vi "MainForKeithley.vi"() -> ()   [LabVIEW 2018]
uses:
  classes/Tushars Events Toolkit/Software/Modules/EventClient_ObjectReference.ctl
  classes/Variable Manager/VariableManager_Bool.vi
  classes/Variable Manager/VariableManager_Double.vi
  <vilib>/Utility/file.llb/Write To Spreadsheet File (string).vi
  classes/Variable Manager/VariableManager_String.vi
  Strict Type Controls/Command.ctl
panel:
  out "filterSetup?":bool
  out "Quit":bool
  out "error out":errorcluster
  in  "error in (no error)":errorcluster
  in  "abort":bool
  in  "start":bool
  out "gratSetup?":bool
  out "statusFilter":bool
  in  "Start Filter":bool
  out "Agilent Current":dbl format="%#.4f A"
  out "Agilent Voltage":dbl format="%#.4f V"
  out "Test Status":bool
  out "statusMerlin":bool
  out "statusMC":bool
  out "statusPS":bool
  out "statusSM":bool
  in  "Start Merlin":bool
  in  "Start Monochromator":bool
  in  "Start Power Supply":bool
  in  "Start Source Meter":bool
  out "Merlin Voltage":dbl format="%#.7f mV"
  out "Measuring Wavelength":dbl format="%#.7f nm"
  out "Source Meter Voltage":dbl format="%#.7f mV"
  in  "tab":T1(tab)=enum."Script"
  in  "exportVT":bool
  out "VTGraph":cluster{dbl[], dbl[]}(graph)
  in  "Test Mode":enum16{"Time Mode", "dV/dt Mode"}(ring)
  in  "Log Interval":u32=50 min=100 step=1 format="%.0f mSec"
  in  "Test Time":dbl step=1.0 format="%<%H:%M:%S>t"
  out "Time Remaining":dbl format="%<%H:%M:%S>t"
  in  "Target dV/dt":dbl format="%#.9f mV"
  in  "Lock In time":dbl step=1.0 format="%<%H:%M:%S>t"
  out "dV/dt":dbl format="%#.11f mV"
  out "Locked Time":dbl step=1.0 format="%<%H:%M:%S>t"
  in  "Perform Test After":T1(ring)=enum."Voltage Vs Wavelength"
  in  "Frequency":u32=8 min=8 max=1100 step=1
  in  "setOffsets":bool
  in  "portD":bool
  in  "portA":bool
  in  "Settling Time (ms)":dbl=5000.0
  in  "To":dbl=1000.0
  in  "Step":dbl=100.0
  in  "From":dbl=100.0
  in  "exportSweep":bool
  out "sweep":cluster{dbl[], dbl[]}[](graph)
  in  "SetSlit":bool
  in  "SetGrating":bool
  in  "setWavelength":bool
  in  "Wavelength":dbl
  in  "Slit":string(combo)
  in  "GratingNo":u8=1 min=1 max=3 step=1
  in  "setMerlin":bool
  in  "#Filter Stages":enum16{"None", "1 Pole", "2 Pole"}(ring)
  in  "Phase":enum16{"1 Phase", "2 Phase"}(ring)
  in  "SyncMode":T2(ring)
  in  "Time Const":T3(ring)
  in  "Sweep Results":i32(listbox)
  in  "tabOnScript":enum32{"V Vs Time", "V Vs Wavelength"}(tab)
  out "scriptGraph":cluster{dbl[], dbl[]}(graph)
  in  "exportScriptResults":bool
  out "scriptSweep":cluster{dbl[], dbl[]}[](graph)
  in  "exportScriptWave":bool
  in  "Command":T4
  in  "Parm 4":dbl format="%#.6f"
  in  "Parm 3":dbl format="%#.6f"
  in  "openScript":bool
  in  "exportScript":bool
  in  "update":bool
  in  "Parm 2":dbl format="%#.6f"
  in  "Parm 1":dbl format="%#.6f"
  in  "script":i32(listbox)
  in  "add":bool
  in  "remove":bool
  in  "Script Avg Interval":u32=200 min=100 step=1 format="%.0f mSec"
  # "Status"
  # "Test Type"
  # "Test Time"
  # "Voltage Results"
  # "Monochromator"
  # "Sweep"
  # "NOTE:\n1. if this LED is OFF then GPIB is not connected...\n2. Close program before power off Instruments..."
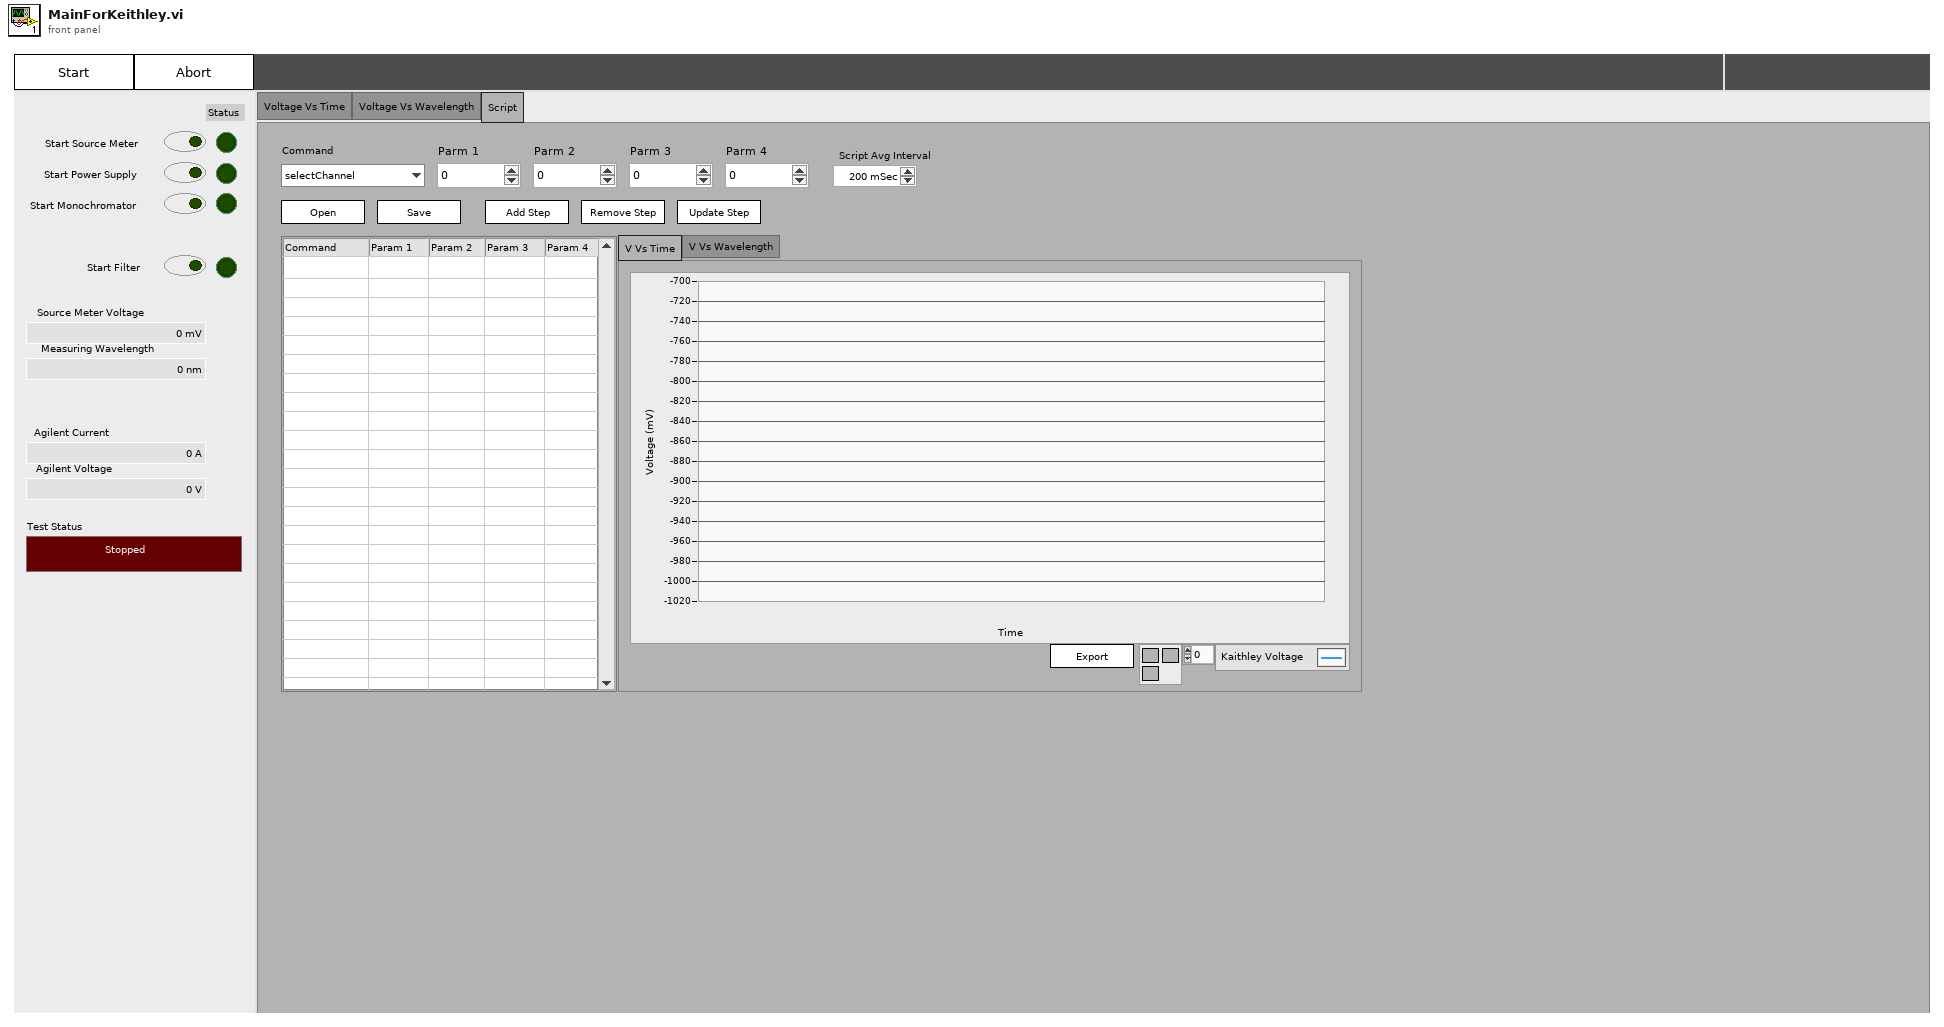
[diagram p1: front panel]
types:
  T1 = enum32{"Voltage Vs Time", "Voltage Vs Wavelength", "Script"}
  T2 = enum16{"Int Chop Off", "Int Chop On", "Ext Chop Off", "Ext Chop On"}
  T3 = enum16{".003s", ".010s", ".030s", ".100s", ".300s", "1.00s", "3.00s", "10.0s", "30.0s", "100s"}
  T4 = typedef "Command.ctl" = enum16{"selectChannel", "setDCVoltage", "setDCCurrent", "setVoltageSteps", "wait", "setWavelength", "setWavelengthSteps"}
  T5 = enum32{"invalid app kind", "Development System", "Run Time System", "Student Edition", "Embedded LabVIEW", "Evaluation", "Custom"}
  T6 = cluster{"startTime":u32, "lastUpdate":u32, "lastVoltage":dbl, "run?":bool, "From":dbl, "time":dbl[], "MerlinVal":dbl[], "SMVolt":dbl[], "sweepType":enum16{"ASC", "DESC"}, "Wavlnth":dbl[], "Test Mode":enum16{"Time Mode", "dV/dt Mode"}, "tab":enum32{"Voltage Vs Time", "Voltage Vs Wavelength", "Script"}, "script":string[][], "dV/dt":dbl[], "graphUpdate":u32}
  T7 = typedef "EventClient_ObjectReference.ctl" = refnum<k1>
  T8 = cluster{"#Stages":enum16{"None", "1 Pole", "2 Pole"}, "Phase":enum16{"1 Phase", "2 Phase"}, "SyncMode":enum16{"Int Chop Off", "Int Chop On", "Ext Chop Off", "Ext Chop On"}, "Time Const":enum16{".003s", ".010s", ".030s", ".100s", ".300s", "1.00s", "3.00s", "10.0s", "30.0s", "100s"}, "Frequency":u32}
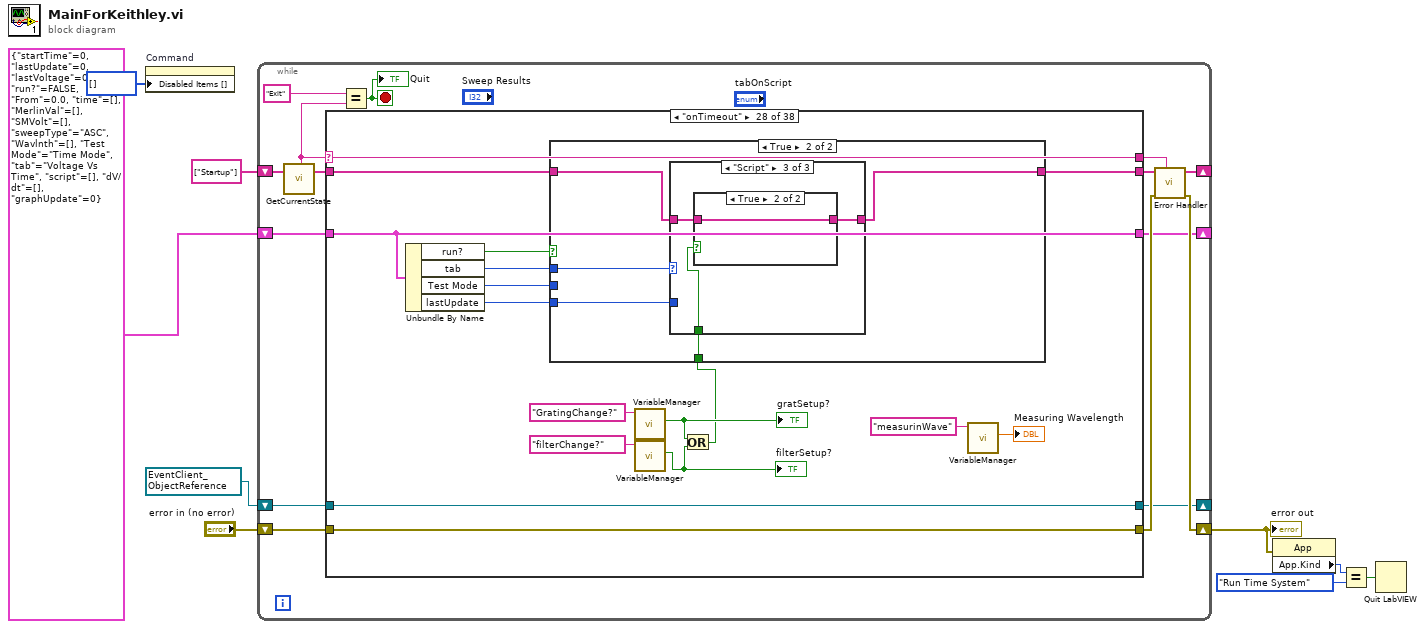
[diagram p0: block diagram]
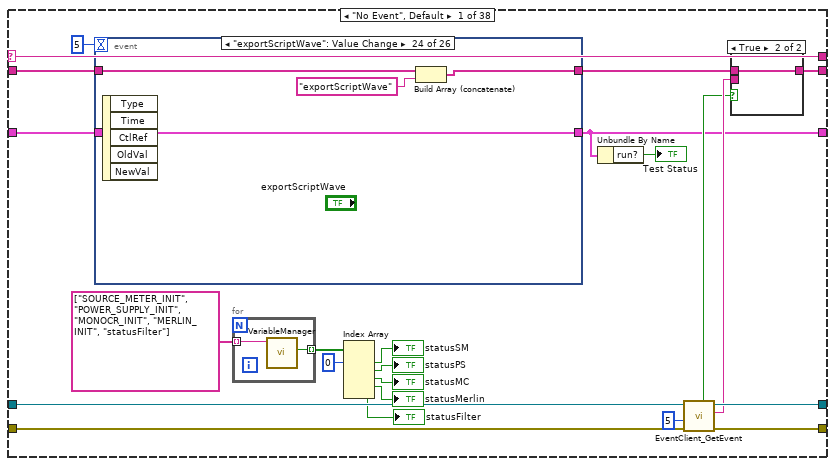
[diagram p2: hidden frame]
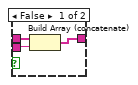
[diagram p3: hidden frame]
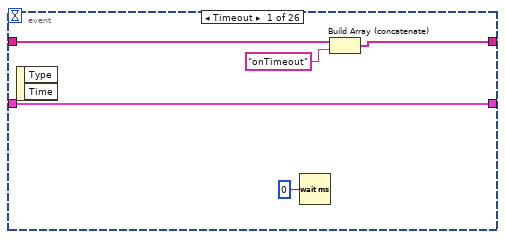
[diagram p4: hidden frame]
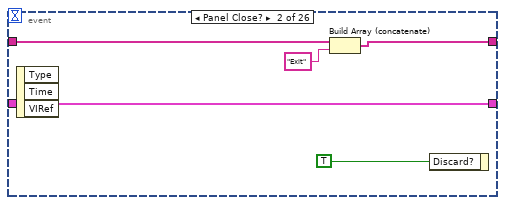
[diagram p5: hidden frame]
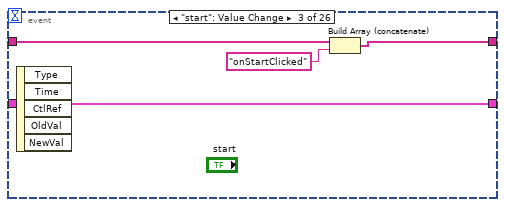
[diagram p6: hidden frame]
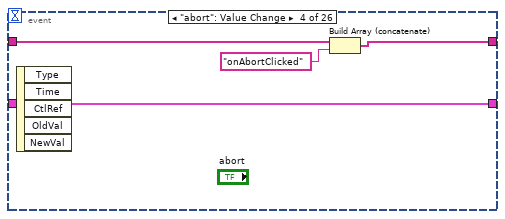
[diagram p7: hidden frame]
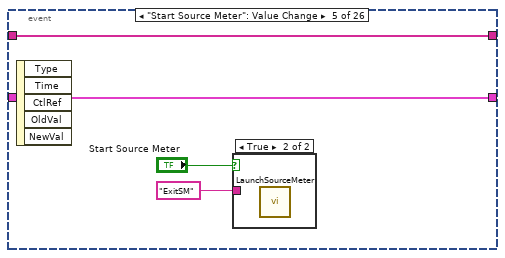
[diagram p8: hidden frame]
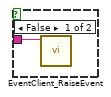
[diagram p9: hidden frame]
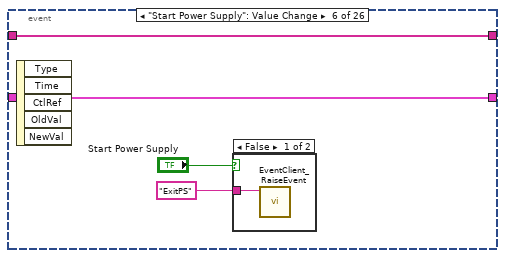
[diagram p10: hidden frame]
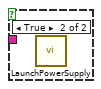
[diagram p11: hidden frame]
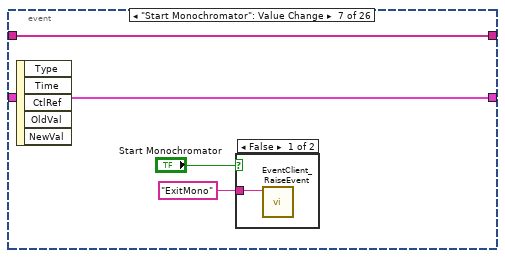
[diagram p12: hidden frame]
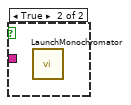
[diagram p13: hidden frame]
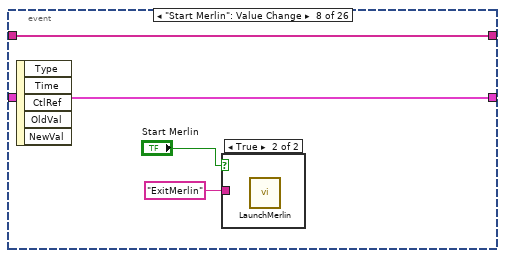
[diagram p14: hidden frame]
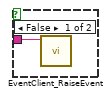
[diagram p15: hidden frame]
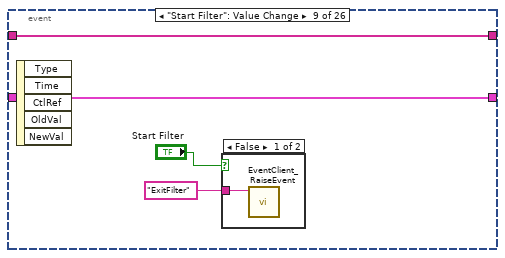
[diagram p16: hidden frame]
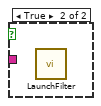
[diagram p17: hidden frame]
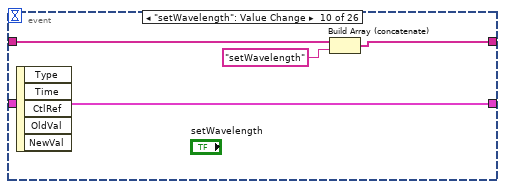
[diagram p18: hidden frame]
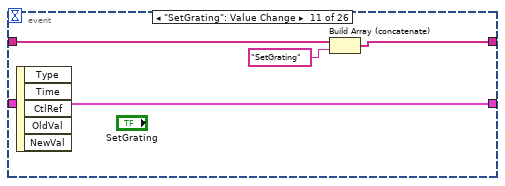
[diagram p19: hidden frame]
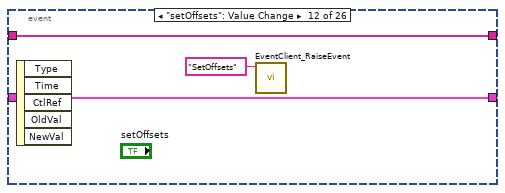
[diagram p20: hidden frame]
diagram:
  w8 = T7 refnum items=["EventClient"] ("reference")
  n1 = property on="Command" class="Enum (strict)"("Disabled Items []"=i32[] []) -> ()  [unwired: 2 in, 2 out]
  n2 = while {
    shift-right: [w20] -> _
    shift-left: string[] ["Startup"] ("State Array Out") -> [w24]
    shift-right: [w16] -> w5
    shift-left: "error in (no error)" -> [w17]
    shift-right: [w13] -> _
    shift-left: w8 -> [w12]
    shift-right: [w10] -> _
    shift-left: T6 {"startTime"=0, "lastUpdate"=0, "lastVoltage"=0.0, "run?"=FALSE, "From"=0.0, "time"=[], "MerlinVal"=[], "SMVolt"=[], "sweepType"=enum."ASC", "Wavlnth"=[], "Test Mode"=enum."Time Mode", "tab"=enum."Voltage Vs Time", "script"=[], "dV/dt"=[], "graphUpdate"=0} -> [w11]
    stop <- w21 stop-if-true
    n3 = call "GetCurrentState.vi"("State Array In"=w24) -> ("Current State"=w14:string, "State Array Out"=w23:string[])  [unwired: 17 in]
    n4 = case shown="\"onTimeout\"" w14 {
      selector: w14 -> [w47 w189 w198 w208 w226 w242 w265 w292 w310 w321 w342 w359 w367 w394 w410 w421 w433 w441 w445 w454 w463 w475 w483 w493 w522 w533 w538 w556 w608 w628 w658 w690 w715 w779 w834 w869 w898 w914]
      tunnel: w23 -> [w46 w188 w204 w209 w227 w243 w266 w293 w311 w322 w343 w360 w368 w395 w411 w422 w434 w442 w449 w458 w465 w479 w484 w494 w523 w534 w539 w547 w591 w612 w650 w682 w706 w780 w835 w870 w897 w901]
      tunnel: [w37 w187 w204 w209 w227 w243 w266 w293 w311 w322 w343 w360 w368 w395 w411 w422 w434 w442 w449 w458 w465 w479 w484 w494 w523 w534 w539 w548 w590 w611 w649 w684 w705 w780 w823 w870 w897 w901] -> w19
      tunnel: [w42 w181 w199 w207 w225 w241 w264 w291 w309 w320 w341 w358 w366 w393 w409 w420 w427 w435 w446 w455 w461 w476 w482 w489 w518 w529 w537 w555 w607 w627 w657 w689 w713 w761 w830 w868 w896 errorcluster {"status"=FALSE, "code"=0, "source"=""} ("error in (no error)")] -> w15
      tunnel: [w47 w189 w198 w208 w226 w242 w265 w292 w310 w321 w342 w359 w367 w394 w410 w421 w433 w441 w445 w454 w463 w475 w483 w493 w522 w533 w538 w556 w608 w628 w658 w690 w715 w779 w834 w869 w898 w914] -> w18
      tunnel: w17 -> [w43 w168 w202 w207 w225 w241 w264 w291 w309 w320 w341 w358 w366 w393 w409 w420 w428 w436 w447 w456 w460 w477 w482 w491 w520 w531 w537 w555 w607 w627 w657 w689 w713 w760 w831 w868 w896 w902]
      tunnel: [w41 w179 w201 w206 w224 w240 w263 w290 w308 w319 w340 w357 w365 w392 w408 w419 w432 w440 w448 w457 w464 w478 w481 w487 w516 w527 w536 w554 w606 w626 w656 w688 w714 w778 w833 w867 w895 w900] -> w13
      tunnel: w12 -> [w44 _ w203 w206 w224 w240 w263 w290 w308 w319 w340 w357 w365 w392 w408 w419 w432 w440 w448 w457 w464 w478 w481 w492 w521 w532 w536 w554 w606 w626 w656 w688 w714 w778 w833 w867 w895 w900]
      tunnel: w11 -> [w28 w177 w197 w205 w223 w239 w262 w289 w307 w318 w339 w356 w364 w391 w407 w418 w431 w439 w443 w453 w462 w468 w480 w485 w515 w526 w535 w553 w596 w625 w654 w687 w708 w777 w821 w860 w894 w899]
      tunnel: [w27 w177 w197 w205 w223 w239 w262 w289 w307 w318 w339 w356 w364 w390 w406 w418 w431 w439 w443 w453 w462 w468 w480 w485 w515 w526 w535 w553 w595 w622 w652 w687 w707 w776 w832 w859 w894 w899] -> w10
      frame "No Event", Default {
        n5 = event shown="[23] \"exportScriptWave\": Value Change" {
          selector: _ -> [_ _ _ _ _ _ _ _ _ _ _ _ _ _ _ _ _ _ _ _ _ _ _ _ _ _]
          dyn-events: _ -> [_ _ _ _ _ _ _ _ _ _ _ _ _ _ _ _ _ _ _ _ _ _ _ _ _ _]
          timeout: 5 -> [_ _ _ _ _ _ _ _ _ _ _ _ _ _ _ _ _ _ _ _ _ _ _ _ _ _]
          tunnel: [w56 w61 w66 w70 w75 w80 w85 w90 w95 w99 w103 w106 w110 w114 w118 w122 w126 w130 w134 w138 w142 w146 w150 w154 w158 w162] -> w38
          tunnel: w46 -> [w58 w63 w67 w71 w75 w80 w85 w90 w95 w100 w104 w106 w111 w115 w119 w123 w127 w131 w135 w139 w143 w147 w151 w155 w159 w163]
          tunnel: w28 -> [w57 w59 w64 w68 w74 w79 w84 w89 w94 w97 w101 w107 w108 w112 w116 w120 w124 w128 w132 w136 w140 w144 w148 w152 w156 w160]
          tunnel: [w57 w59 w64 w68 w74 w79 w84 w89 w94 w97 w101 w107 w108 w112 w116 w120 w124 w128 w132 w136 w140 w144 w148 w152 w156 w160] -> w27
          event Timeout {
            n6 = event-data() -> ()  [unwired: 1 in, 2 out]
            n7 = Wait (ms)(milliseconds to wait=u32 0) -> ()  [unwired: 1 out]
            n8 = Build Array (concatenate)(w58, "onTimeout" ("x")) -> (w56:string[])
          }
          event Panel Close? {
            n9 = event-data() -> ()  [unwired: 1 in, 3 out]
            n10 = Build Array (concatenate)(w63, "Exit" ("x")) -> (w61:string[])
            n11 = event-data("Discard?"=TRUE) -> ()  [unwired: 1 in, 1 out]
          }
          event "start": Value Change {
            n12 = event-data() -> ()  [unwired: 1 in, 5 out]
            n13 = Build Array (concatenate)(w67, "onStartClicked" ("x")) -> (w66:string[])
          }
          event "abort": Value Change {
            n14 = event-data() -> ()  [unwired: 1 in, 5 out]
            n15 = Build Array (concatenate)(w71, "onAbortClicked" ("x")) -> (w70:string[])
          }
          event "Start Source Meter": Value Change {
            n16 = event-data() -> ()  [unwired: 1 in, 5 out]
            n17 = case shown="True" "Start Source Meter" {
              tunnel: "ExitSM" -> [w76 _]
              frame False {
                n18 = call "EventClient_RaiseEvent.vi"("Event"=w76) -> ()  [unwired: 10 in, 1 out]
              }
              frame True {
                n19 = call "LaunchSourceMeter.vi"() -> ()  [unwired: 11 in, 1 out]
              }
            }
          }
          event "Start Power Supply": Value Change {
            n20 = event-data() -> ()  [unwired: 1 in, 5 out]
            n21 = case shown="False" "Start Power Supply" {
              tunnel: "ExitPS" -> [w81 _]
              frame False {
                n22 = call "EventClient_RaiseEvent.vi"("Event"=w81) -> ()  [unwired: 10 in, 1 out]
              }
              frame True {
                n23 = call "LaunchPowerSupply.vi"() -> ()  [unwired: 11 in, 1 out]
              }
            }
          }
          event "Start Monochromator": Value Change {
            n24 = event-data() -> ()  [unwired: 1 in, 5 out]
            n25 = case shown="False" "Start Monochromator" {
              tunnel: "ExitMono" -> [w86 _]
              frame False {
                n26 = call "EventClient_RaiseEvent.vi"("Event"=w86) -> ()  [unwired: 10 in, 1 out]
              }
              frame True {
                n27 = call "LaunchMonochromator.vi"() -> ()  [unwired: 11 in, 1 out]
              }
            }
          }
          event "Start Merlin": Value Change {
            n28 = event-data() -> ()  [unwired: 1 in, 5 out]
            n29 = case shown="True" "Start Merlin" {
              tunnel: "ExitMerlin" -> [w91 _]
              frame False {
                n30 = call "EventClient_RaiseEvent.vi"("Event"=w91) -> ()  [unwired: 10 in, 1 out]
              }
              frame True {
                n31 = call "LaunchMerlin.vi"() -> ()  [unwired: 11 in, 1 out]
              }
            }
          }
          event "Start Filter": Value Change {
            n32 = event-data() -> ()  [unwired: 1 in, 5 out]
            n33 = case shown="False" "Start Filter" {
              tunnel: "ExitFilter" -> [w96 _]
              frame False {
                n34 = call "EventClient_RaiseEvent.vi"("Event"=w96) -> ()  [unwired: 10 in, 1 out]
              }
              frame True {
                n35 = call "LaunchFilter.vi"() -> ()  [unwired: 11 in, 1 out]
              }
            }
          }
          event "setWavelength": Value Change {
            n36 = event-data() -> ()  [unwired: 1 in, 5 out]
            n37 = Build Array (concatenate)(w100, "setWavelength" ("x")) -> (w99:string[])
          }
          event "SetGrating": Value Change {
            n38 = event-data() -> ()  [unwired: 1 in, 5 out]
            n39 = Build Array (concatenate)(w104, "SetGrating" ("x")) -> (w103:string[])
          }
          event "setOffsets": Value Change {
            n40 = event-data() -> ()  [unwired: 1 in, 5 out]
            n41 = call "EventClient_RaiseEvent.vi"("Event"="SetOffsets") -> ()  [unwired: 10 in, 1 out]
          }
          event "SetSlit": Value Change {
            n42 = event-data() -> ()  [unwired: 1 in, 5 out]
            n43 = Build Array (concatenate)(w111, "SetSlit" ("x")) -> (w110:string[])
          }
          event "setMerlin": Value Change {
            n44 = event-data() -> ()  [unwired: 1 in, 5 out]
            n45 = Build Array (concatenate)(w115, "setMerlin" ("x")) -> (w114:string[])
          }
          event "exportSweep": Value Change {
            n46 = event-data() -> ()  [unwired: 1 in, 5 out]
            n47 = Build Array (concatenate)(w119, "exportSweep" ("x")) -> (w118:string[])
          }
          event "exportVT": Value Change {
            n48 = event-data() -> ()  [unwired: 1 in, 5 out]
            n49 = Build Array (concatenate)(w123, "exportVT" ("x")) -> (w122:string[])
          }
          event "portA": Value Change {
            n50 = event-data() -> ()  [unwired: 1 in, 5 out]
            n51 = Build Array (concatenate)(w127, "portA" ("x")) -> (w126:string[])
          }
          event "portD": Value Change {
            n52 = event-data() -> ()  [unwired: 1 in, 5 out]
            n53 = Build Array (concatenate)(w131, "portD" ("x")) -> (w130:string[])
          }
          event "add": Value Change {
            n54 = event-data() -> ()  [unwired: 1 in, 5 out]
            n55 = Build Array (concatenate)(w135, "addStep" ("x")) -> (w134:string[])
          }
          event "remove": Value Change {
            n56 = event-data() -> ()  [unwired: 1 in, 5 out]
            n57 = Build Array (concatenate)(w139, "removeStep" ("x")) -> (w138:string[])
          }
          event "update": Value Change {
            n58 = event-data() -> ()  [unwired: 1 in, 5 out]
            n59 = Build Array (concatenate)(w143, "updateStep" ("x")) -> (w142:string[])
          }
          event "exportScript": Value Change {
            n60 = event-data() -> ()  [unwired: 1 in, 5 out]
            n61 = Build Array (concatenate)(w147, "exportScript" ("x")) -> (w146:string[])
          }
          event "exportScriptResults": Value Change {
            n62 = event-data() -> ()  [unwired: 1 in, 5 out]
            n63 = Build Array (concatenate)(w151, "exportScriptResults" ("x")) -> (w150:string[])
          }
          event "exportScriptWave": Value Change {
            n64 = event-data() -> ()  [unwired: 1 in, 5 out]
            n65 = Build Array (concatenate)(w155, "exportScriptWave" ("x")) -> (w154:string[])
          }
          event "openScript": Value Change {
            n66 = event-data() -> ()  [unwired: 1 in, 5 out]
            n67 = Build Array (concatenate)(w159, "openScript" ("x")) -> (w158:string[])
          }
          event "script": Value Change {
            n68 = event-data() -> ()  [unwired: 1 in, 5 out]
            n69 = Build Array (concatenate)(w163, "onScriptRowSelected" ("x")) -> (w162:string[])
          }
        }
        n70 = for {
          tunnel: string[] ["SOURCE_METER_INIT", "POWER_SUPPLY_INIT", "MONOCR_INIT", "MERLIN_INIT", "statusFilter"] ("State Array Out") -> [w49] mode=indexing
          tunnel: [w48] -> w34 mode=indexing
          n71 = call-poly "VariableManager.vi"("Tag"=w49) -> ("Value out"=w48:bool)  [unwired: 7 in, 3 out]
        }
        n72 = Index Array(array=w34, index #1=0 ("index")) -> (element #1=→"statusSM":bool, element #2=→"statusPS":bool, element #3=→"statusMC":bool, element #4=→"statusMerlin":bool, element #5=→"statusFilter":bool)  [unwired: 4 in]
        n73 = Unbundle By Name(w27) -> ("run?"=→"Test Status":bool)
        n74 = call "EventClient_GetEvent.vi"("error in (no error)"=w43, "timeout in ms (-1)"=5, "reference"=w44) -> ("error out"=w42:errorcluster, "Name"=w40:string, "reference out"=w41:T7, "timed out?"=w39:bool)  [unwired: 4 in, 1 out]
        n75 = case shown="True" w39 {
          tunnel: w38 -> [w52 w53]
          tunnel: w40 -> [w51 _]
          tunnel: [w50 w53] -> w37
          frame False {
            n76 = Build Array (concatenate)(w52, w51) -> (w50:string[])
          }
          frame True {
          }
        }
      }
      frame "Startup" {
        w166 = cluster{dbl[], dbl[]}[] [] ("sweep")
        w167 = cluster{dbl[], dbl[]} {[], []} ("VTGraph")
        w171 = string[] ["Command", "Param 1", "Param 2", "Param 3", "Param 4"]  # script
        w172 = FALSE ("Start Source Meter")
        w165 = u32 200 ("Log Interval")
        # "If Multiple instnances of this VI are possible \nthen make sure that client created in each instance gets a different Name"
        n77 = local write "Log Interval"(w165) -> ()
        n78 = local write "Target dV/dt"(1.0 ("Target dV/dt")) -> ()
        n79 = local write "Lock In time"(30.0 ("Lock In time")) -> ()
        n80 = local write "sweep"(w166) -> ()
        n81 = local write "Test Time"(90.0 ("Locked Time")) -> ()
        n82 = local write "VTGraph"(w167) -> ()
        n83 = local write "scriptGraph"(w167) -> ()
        n84 = local write "Script Avg Interval"(w165) -> ()
        n85 = disable-structure shown="Disabled" {
          disable-tunnel: [w196 _] -> w173
          disable-tunnel: w168 -> [w195 _]
          frame Disabled {
            n86 = call "LaunchPowerSupply.vi"("error in (no error)"=w195) -> ("error out"=w194:errorcluster)  [unwired: 10 in]
            n87 = call "LaunchSourceMeter.vi"("error in (no error)"=w194) -> ("error out"=w193:errorcluster)  [unwired: 10 in]
            n88 = call "LaunchMerlin.vi"("error in (no error)"=w193) -> ("error out"=w192:errorcluster)  [unwired: 10 in]
            n89 = call "LaunchMonochromator.vi"("error in (no error)"=w192) -> ("error out"=w196:errorcluster)  [unwired: 10 in]
          }
          frame Enabled {
          }
        }
        n90 = local write "scriptSweep"(w166) -> ()
        n91 = local write "tab"(T1."Voltage Vs Wavelength" ("tab")) -> ()
        n92 = for {
          tunnel: bool[] [TRUE, FALSE] -> [w190] mode=indexing
          i -> [w191]
          n93 = property on="sweep" class="XYGraph (strict)"("Active Plot"=w191, "Plot.Visible?"=w190) -> ()  [unwired: 2 in, 2 out]
          n94 = property on="scriptSweep" class="XYGraph (strict)"("Active Plot"=w191, "Plot.Visible?"=w190) -> ()  [unwired: 2 in, 2 out]
        }
        n95 = Build Array (concatenate)(w188, string[] [] ("State Array Out")) -> (w187:string[])
        n96 = Call Chain() -> (call chain=w185:string[])
        n97 = Index Array(array=w185, index=0) -> (element=w183:string)
        n98 = call "EventClient_Create.vi"("error in (no error)"=w173, "Instance Name"=w183) -> ("error out"=w182:errorcluster, "reference"=w180:T7)  [unwired: 8 in]
        n99 = local write "Start Source Meter"(w172) -> ()
        n100 = local write "Start Power Supply"(w172) -> ()
        n101 = local write "Start Monochromator"(w172) -> ()
        n102 = local write "Start Merlin"(w172) -> ()
        n103 = call "EventClient_SubscribeEvents.vi"("error in (no error)"=w182, "Events"=string[] ["currGrating", "updateScriptSweep"], "reference"=w180) -> ("error out"=w181:errorcluster, "reference out"=w179:T7)  [unwired: 7 in]
        n104 = property on="script" class="MCListbox (strict)"("ColHdrString"=w171, "ItemNames"=string[][] [] ("Item Names")) -> ()  [unwired: 2 in, 2 out]
      }
      frame "Exit" {
        w201 = T7 refnum items=["EventClient"] ("reference out")
        n105 = call "EventClient_Destroy.vi"("error in (no error)"=w202, "reference"=w203) -> ("error out"=w200:errorcluster)  [unwired: 9 in]
        n106 = call "EventClient_RaiseEvent.vi"("error in (no error)"=w200, "Event"=w198) -> ("error out"=w199:errorcluster)  [unwired: 9 in]
      }
      frame "---------------Below are UI Events---------------" {
        # "This State will never Execute\nIt is added just for improving code readability please do not remove this case"
      }
      frame "onScriptRowSelected" {
        w215 = 0 ("index")
        n107 = property on="script" class="MCListbox (strict)"() -> ("ItemNames"=w222:string[][], "Value"=w221:i32)  [unwired: 2 in, 2 out]
        n108 = Index Array(array=w222, index (row)=w221) -> (element=w219:string[])  [unwired: 1 in]
        n109 = Delete From Array(array=w219, index=w215) -> (deleted portion=w218:string, array with subset deleted=w220:string[])  [unwired: 1 in]
        n110 = Scan From String(input string=w218, default 1=Command."selectChannel" ("Command")) -> (output 1=w214:T4)  [unwired: 3 in, 3 out]
        n111 = Fract/Exp String To Number(string=w220) -> (number=w216:dbl[])  [unwired: 3 in, 1 out]
        n112 = Index Array(array=w216, index #1=w215) -> (element #1=w213:dbl, element #2=w212:dbl, element #3=w211:dbl, element #4=w210:dbl)  [unwired: 3 in]
        n113 = local write "Parm 1"(w213) -> ()
        n114 = local write "Parm 2"(w212) -> ()
        n115 = local write "Parm 3"(w211) -> ()
        n116 = local write "Parm 4"(w210) -> ()
        n117 = local write "Command"(w214) -> ()
      }
      frame "exportVT" {
        n118 = local read "VTGraph"() -> (w233:cluster{dbl[], dbl[]})
        n119 = Unbundle(w233) -> (w237:dbl[], w234:dbl[])
        n120 = for {
          tunnel: w237 -> [w248] mode=indexing
          tunnel: "%<%H:%M:%S>t" ("format string") -> [w250]
          tunnel: [w249] -> w236 mode=indexing
          n121 = Format Into String(format string=w250, w248) -> (resulting string=w249:string)  [unwired: 2 in, 1 out]
        }
        n122 = Number To Fractional String(number=w234) -> (F-format string=w235:string[])  [unwired: 3 in]
        n123 = Build Array(w236, w235) -> (w232:string[][])
        n124 = Transpose 2D Array(2D array=w232) -> (transposed array=w228:string[][])
        n125 = call "File Dialog2"("pattern (all files)"="*.csv") -> ("selected path"=w231:path, "error out"=w230:errorcluster)  [unwired: 11 in, 2 out]
        n126 = case shown="Error" w230 {
          selector: w230 -> [_ w247]
          tunnel: w231 -> [w245 _]
          tunnel: w228 -> [w244 _]
          frame No Error {
            n127 = call-poly <vilib>:"Write To Spreadsheet File.vi"("delimiter (\\t)"="," ("delimiter (\\t)"), "2D data"=w244, "file path (dialog if empty)"=w245) -> ()  [unwired: 5 in, 1 out]
          }
          frame Error {
            n128 = call <vilib>:"Clear Errors.vi"("error in (no error)"=w247) -> ()  [unwired: 5 in, 2 out]
          }
        }
      }
      frame "exportScriptResults" {
        n129 = local read "scriptGraph"() -> (w257:cluster{dbl[], dbl[]})
        n130 = Unbundle(w257) -> (w260:dbl[], w256:dbl[])
        n131 = for {
          tunnel: w260 -> [w271] mode=indexing
          tunnel: "%<%H:%M:%S>t" ("format string") -> [w273]
          tunnel: [w272] -> w259 mode=indexing
          n132 = Format Into String(format string=w273, w271) -> (resulting string=w272:string)  [unwired: 2 in, 1 out]
        }
        n133 = Number To Fractional String(number=w256) -> (F-format string=w258:string[])  [unwired: 3 in]
        n134 = Build Array(w259, w258) -> (w255:string[][])
        n135 = Transpose 2D Array(2D array=w255) -> (transposed array=w251:string[][])
        n136 = call "File Dialog3"("pattern (all files)"="*.csv") -> ("selected path"=w254:path, "error out"=w253:errorcluster)  [unwired: 11 in, 2 out]
        n137 = case shown="No Error" w253 {
          selector: w253 -> [_ w270]
          tunnel: w254 -> [w268 _]
          tunnel: w251 -> [w267 _]
          frame No Error {
            n138 = call-poly <vilib>:"Write To Spreadsheet File.vi"("delimiter (\\t)"="," ("delimiter (\\t)"), "2D data"=w267, "file path (dialog if empty)"=w268) -> ()  [unwired: 5 in, 1 out]
          }
          frame Error {
            n139 = call <vilib>:"Clear Errors.vi"("error in (no error)"=w270) -> ()  [unwired: 5 in, 2 out]
          }
        }
      }
      frame "exportScriptWave" {
        (unwired) "%<%H:%M:%S>t" ("format string")
        n140 = local read "scriptSweep"() -> (w286:cluster{dbl[], dbl[]}[])
        n141 = Index Array(array=w286, index #1=0 ("index")) -> (element #1=w285:cluster{dbl[], dbl[]}, element #2=w283:cluster{dbl[], dbl[]})  [unwired: 1 in]
        n142 = Unbundle(w283) -> (w282:dbl[])  [unwired: 1 out]
        n143 = Unbundle(w285) -> (w274:dbl[], w276:dbl[])
        n144 = Number To Fractional String(number=w274) -> (F-format string=w275:string[])  [unwired: 3 in]
        n145 = Number To Fractional String(number=w276) -> (F-format string=w288:string[])  [unwired: 3 in]
        n146 = Number To Fractional String(number=w282) -> (F-format string=w281:string[])  [unwired: 3 in]
        n147 = Build Array(w275, w288, w281) -> (w287:string[][])
        n148 = Transpose 2D Array(2D array=w287) -> (transposed array=w277:string[][])
        n149 = call "File Dialog4"("pattern (all files)"="*.csv") -> ("selected path"=w280:path, "error out"=w279:errorcluster)  [unwired: 11 in, 2 out]
        n150 = case shown="No Error" w279 {
          selector: w279 -> [_ w297]
          tunnel: w280 -> [w295 _]
          tunnel: w277 -> [w294 _]
          frame No Error {
            n151 = call-poly <vilib>:"Write To Spreadsheet File.vi"("delimiter (\\t)"="," ("delimiter (\\t)"), "2D data"=w294, "file path (dialog if empty)"=w295) -> ()  [unwired: 5 in, 1 out]
          }
          frame Error {
            n152 = call <vilib>:"Clear Errors.vi"("error in (no error)"=w297) -> ()  [unwired: 5 in, 2 out]
          }
        }
      }
      frame "openScript" {
        w302 = string[][] []  # script
        n153 = Read from Text File() -> (text=w305:string, error out=w298:errorcluster)  [unwired: 4 in, 2 out]
        n154 = Spreadsheet String To Array(delimiter (Tab)=",", format string="%s", spreadsheet string=w305, array type (2D Dbl)=w302) -> (array=w301:string[][])
        n155 = call <vilib>:"Clear Errors.vi"("error in (no error)"=w298) -> ()  [unwired: 5 in, 2 out]
        n156 = Delete From Array(array=w301, index (row)=0) -> (deleted portion=w299:string[], array with subset deleted=w300:string[][])  [unwired: 2 in]
        n157 = property on="script" class="MCListbox (strict)"("ItemNames"=w300, "ColHdrString"=w299) -> ()  [unwired: 2 in, 2 out]
      }
      frame "exportScript" {
        n158 = property on="script" class="MCListbox (strict)"() -> ("ColHdrString"=w317:string[], "ItemNames"=w316:string[][])  [unwired: 2 in, 2 out]
        n159 = Build Array (concatenate)(w317, w316) -> (w312:string[][])
        n160 = call "File Dialog5"("pattern (all files)"="*.csv") -> ("selected path"=w315:path, "error out"=w314:errorcluster)  [unwired: 11 in, 2 out]
        n161 = case shown="No Error" w314 {
          selector: w314 -> [_ w326]
          tunnel: w315 -> [w324 _]
          tunnel: w312 -> [w323 _]
          frame No Error {
            n162 = call-poly <vilib>:"Write To Spreadsheet File.vi"("delimiter (\\t)"="," ("delimiter (\\t)"), "2D data"=w323, "file path (dialog if empty)"=w324) -> ()  [unwired: 5 in, 1 out]
          }
          frame Error {
            n163 = call <vilib>:"Clear Errors.vi"("error in (no error)"=w326) -> ()  [unwired: 5 in, 2 out]
          }
        }
      }
      frame "addStep" {
        n164 = property on="script" class="MCListbox (strict)"() -> ("ItemNames"=w336:string[][])  [unwired: 2 in, 2 out]
        n165 = Format Into String("Command") -> (resulting string=w332:string)  [unwired: 3 in, 1 out]
        n166 = Build Array("Parm 1", "Parm 2", "Parm 3", "Parm 4") -> (w333:dbl[])
        n167 = Number To Fractional String(number=w333, width (-)=i16 3 ("precision (6)")) -> (F-format string=w331:string[])  [unwired: 2 in]
        n168 = Build Array (concatenate)(w332, w331) -> (w330:string[])
        n169 = Build Array (concatenate)(w336, w330) -> (w335:string[][])
        n170 = property on="script" class="MCListbox (strict)"("ItemNames"=w335) -> ()  [unwired: 2 in, 2 out]
      }
      frame "updateStep" {
        n171 = local read "Command"() -> (w349:T4)
        n172 = local read "Parm 1"() -> (w348:dbl)
        n173 = local read "Parm 2"() -> (w347:dbl)
        n174 = local read "Parm 3"() -> (w345:dbl)
        n175 = local read "Parm 4"() -> (w344:dbl)
        n176 = Format Into String(w349) -> (resulting string=w351:string)  [unwired: 3 in, 1 out]
        n177 = Build Array(w348, w347, w345, w344) -> (w352:dbl[])
        n178 = property on="script" class="MCListbox (strict)"() -> ("ItemNames"=w355:string[][], "Value"=w353:i32)  [unwired: 2 in, 2 out]
        n179 = Number To Fractional String(number=w352) -> (F-format string=w350:string[])  [unwired: 3 in]
        n180 = Build Array (concatenate)(w351, w350) -> (w346:string[])
        n181 = Replace Array Subset(array=w355, new element=w346, index (row)=w353) -> (w354:string[][])  [unwired: 1 in]
        n182 = property on="script" class="MCListbox (strict)"("ItemNames"=w354) -> ()  [unwired: 2 in, 2 out]
      }
      frame "removeStep" {
        n183 = property on="script" class="MCListbox (strict)"() -> ("ItemNames"=w363:string[][], "Value"=w361:i32)  [unwired: 2 in, 2 out]
        n184 = Delete From Array(array=w363, index (row)=w361) -> (array with subset deleted=w362:string[][])  [unwired: 2 in, 1 out]
        n185 = property on="script" class="MCListbox (strict)"("ItemNames"=w362) -> ()  [unwired: 2 in, 2 out]
      }
      frame "onStartClicked" {
        w379 = dbl[] [] ("time")
        n186 = local write "Locked Time"(0.0 ("Locked Time")) -> ()
        n187 = local read "tab"() -> (w374:T1)
        n188 = case shown="\"Voltage Vs Wavelength\"" w374 {
          tunnel: [u32 0 u32 0 u32 2000] -> w372
          frame "Voltage Vs Time", Default {
            n189 = local write "VTGraph"(cluster{dbl[], dbl[]} {[], []} ("VTGraph")) -> ()
          }
          frame "Script" {
            n190 = local write "scriptSweep"(cluster{dbl[], dbl[]}[] [] ("scriptSweep")) -> ()
            n191 = local write "scriptGraph"(cluster{dbl[], dbl[]} {[], []} ("scriptGraph")) -> ()
          }
          frame "Voltage Vs Wavelength" {
            n192 = local read "From"() -> (w402:dbl)
            n193 = property on="Sweep Results" class="MCListbox (strict)"("ItemNames"=string[][] [] ("Item Names")) -> ()  [unwired: 2 in, 2 out]
            n194 = local write "sweep"(cluster{dbl[], dbl[]}[] [] ("sweep")) -> ()
            n195 = call "setWavelenght.vi"("wavelength"=w402) -> ()  [unwired: 10 in, 1 out]
          }
        }
        n196 = Wait (ms)(milliseconds to wait=w372) -> ()  [unwired: 1 out]
        n197 = property on="script" class="MCListbox (strict)"() -> ("ItemNames"=w375:string[][])  [unwired: 2 in, 2 out]
        n198 = call-poly "VariableManager.vi"("Operation"=enum16{"Get Tag", "Set Tag"}."Set Tag", "Value"=0.0, "Tag"="measurinWave") -> ()  [unwired: 4 in, 5 out]
        n199 = Less Or Equal?(x="From", y="To") -> (x <= y?=w385:bool)
        n200 = Select(t=enum16{"ASC", "DESC"}."ASC" ("sweepType"), s=w385, f=enum16{"ASC", "DESC"}."DESC" ("sweepType")) -> (s? t:f=w383:enum16{"ASC", "DESC"})
        n201 = Tick Count (ms)() -> (millisecond timer value=w373:u32)
        n202 = call-poly "VariableManager.vi"("Tag"="SM_VOLTAGE" ("String")) -> ("Value out"=w387:dbl)  [unwired: 6 in, 4 out]
        n203 = Bundle By Name(cluster=w391, "graphUpdate"=w373, "startTime"=w373, "lastUpdate"=w373, "run?"=TRUE, "lastVoltage"=w387, "time"=w379, "SMVolt"=w379, "MerlinVal"=w379, "Wavlnth"=w379, "sweepType"=w383, "From"="From", "tab"="tab", "Test Mode"="Test Mode", "script"=w375) -> (w390:T6)
        "Time Remaining" <- "Test Time"
      }
      frame "onAbortClicked" {
        n204 = Bundle By Name(cluster=w407, "run?"=FALSE) -> (w406:T6)
      }
      frame "exportSweep" {
        n205 = property on="Sweep Results" class="MCListbox (strict)"() -> ("ColHdrString"=w416:string[], "ItemNames"=w417:string[][])  [unwired: 2 in, 2 out]
        n206 = Build Array (concatenate)(w416, w417) -> (w412:string[][])
        n207 = call "File Dialog"("pattern (all files)"="*.csv") -> ("selected path"=w415:path, "error out"=w414:errorcluster)  [unwired: 11 in, 2 out]
        n208 = case shown="No Error" w414 {
          selector: w414 -> [_ w426]
          tunnel: w415 -> [w424 _]
          tunnel: w412 -> [w423 _]
          frame No Error {
            n209 = call-poly <vilib>:"Write To Spreadsheet File.vi"("delimiter (\\t)"="," ("delimiter (\\t)"), "2D data"=w423, "file path (dialog if empty)"=w424) -> ()  [unwired: 5 in, 1 out]
          }
          frame Error {
            n210 = call <vilib>:"Clear Errors.vi"("error in (no error)"=w426) -> ()  [unwired: 5 in, 2 out]
          }
        }
      }
      frame "portA" {
        n211 = call "EventClient_RaiseEvent.vi"("error in (no error)"=w428, "Data"="!PORTIN A" ("concatenated string"), "Event"="MerlinWrite") -> ("error out"=w427:errorcluster)  [unwired: 8 in]
      }
      frame "portD" {
        n212 = call "EventClient_RaiseEvent.vi"("error in (no error)"=w436, "Data"="!PORTIN D" ("concatenated string"), "Event"="MerlinWrite") -> ("error out"=w435:errorcluster)  [unwired: 8 in]
      }
      frame "SetGrating" {
        n213 = call "EventClient_RaiseEvent.vi"("error in (no error)"=w447, "Data"="GratingNo", "Event"=w445) -> ("error out"=w446:errorcluster)  [unwired: 8 in]
      }
      frame "SetSlit" {
        n214 = call-poly "VariableManager.vi"("Operation"=enum16{"Get Tag", "Set Tag"}."Set Tag", "Value"="Slit", "Tag"="currSlit") -> ()  [unwired: 5 in, 4 out]
        n215 = call "EventClient_RaiseEvent.vi"("error in (no error)"=w456, "Data"="Slit", "Event"=w454) -> ("error out"=w455:errorcluster)  [unwired: 8 in]
      }
      frame "setWavelength" {
        n216 = call "setWavelenght.vi"("error in (no error)"=w460, "wavelength"="Wavelength") -> ("error out"=w461:errorcluster)  [unwired: 9 in]
      }
      frame "setMerlin" {
        n217 = Bundle By Name(cluster=T8 {"#Stages"=enum."None", "Phase"=enum."1 Phase", "SyncMode"=enum."Int Chop Off", "Time Const"=enum.".003s", "Frequency"=0}, "#Stages"="#Filter Stages", "Phase"="Phase", "SyncMode"="SyncMode", "Time Const"="Time Const", "Frequency"="Frequency") -> (w474:T8)
        n218 = call "EventClient_RaiseEvent.vi"("error in (no error)"=w477, "Data"=w474, "Event"="setMerlin") -> ("error out"=w476:errorcluster)  [unwired: 8 in]
      }
      frame "---------------Below are Menu Events---------------" {
        # "This State will never Execute\nIt is added just for improving code readability please do not remove this case"
      }
      frame "---------------Below are Client Events---------------" {
        # "To Handle Event Duplicate this case. If Event Does not have any data then remove\nGet Event Data and variant to data VIs"
        # "Connect Proper DataType Here"
        n219 = call "EventClient_GetEventData.vi"("error in (no error)"=w491, "reference"=w492) -> ("error out"=w490:errorcluster, "Data"=w488:variant, "reference out"=w487:T7)  [unwired: 7 in]
        n220 = Variant To Data(error in=w490, type=variant, Variant=w488) -> (error out=w489:errorcluster)  [unwired: 1 out]
      }
      frame "updateScriptSweep" {
        n221 = call "EventClient_GetEventData.vi"("error in (no error)"=w520, "reference"=w521) -> ("error out"=w519:errorcluster, "Data"=w517:variant, "reference out"=w516:T7)  [unwired: 7 in]
        n222 = Variant To Data(error in=w519, type=cluster{"wave":dbl, "smV":dbl, "mV":dbl} {"wave"=0.0, "smV"=0.0, "mV"=0.0}, Variant=w517) -> (data=w498:cluster{"wave":dbl, "smV":dbl, "mV":dbl}, error out=w518:errorcluster)
        n223 = local read "scriptSweep"() -> (w500:cluster{dbl[], dbl[]}[])
        n224 = Unbundle By Name(w498) -> ("wave"=w497:dbl, "smV"=w496:dbl, "mV"=w495:dbl)
        n225 = Index Array(array=w500, index #1=0 ("index")) -> (element #1=w502:cluster{dbl[], dbl[]}, element #2=w505:cluster{dbl[], dbl[]})  [unwired: 1 in]
        n226 = Unbundle(w502) -> (w507:dbl[], w508:dbl[])
        n227 = Unbundle(w505) -> (w506:dbl[], w509:dbl[])
        n228 = Build Array (concatenate)(w507, w497) -> (w504:dbl[])
        n229 = Build Array (concatenate)(w508, w496) -> (w512:dbl[])
        n230 = Build Array (concatenate)(w506, w497) -> (w510:dbl[])
        n231 = Build Array (concatenate)(w509, w495) -> (w511:dbl[])
        n232 = Bundle(cluster=w502, w504, w512) -> (w503:cluster{dbl[], dbl[]})
        n233 = Bundle(w510, w511) -> (w513:cluster{dbl[], dbl[]})  [unwired: 1 in]
        n234 = Build Array(w503, w513) -> (→"scriptSweep":cluster{dbl[], dbl[]}[])
      }
      frame "currGrating" {
        n235 = call "EventClient_GetEventData.vi"("error in (no error)"=w531, "reference"=w532) -> ("error out"=w530:errorcluster, "Data"=w528:variant, "reference out"=w527:T7)  [unwired: 7 in]
        n236 = Variant To Data(error in=w530, type=u32 0, Variant=w528) -> (data=w524:u32, error out=w529:errorcluster)
        n237 = local write "GratingNo"(w524) -> ()
      }
      frame "---------------Below are Subroutine states---------------" {
      }
      frame "onTimeout" {
        n238 = Unbundle By Name(w553) -> ("run?"=w552:bool, "tab"=w551:T1, "Test Mode"=w550:enum16{"Time Mode", "dV/dt Mode"}, "lastUpdate"=w549:u32)
        n239 = call-poly "VariableManager.vi"("Tag"="GratingChange?") -> ("Value out"=w544:bool)  [unwired: 7 in, 3 out]
        "gratSetup?" <- w544
        n240 = call-poly "VariableManager.vi"("Tag"="filterChange?") -> ("Value out"=w543:bool)  [unwired: 7 in, 3 out]
        "filterSetup?" <- w543
        n241 = Or(x=w544, y=w543) -> (x .or. y?=w542:bool)
        n242 = case shown="True" w552 {
          tunnel: w551 -> [_ w571]
          tunnel: w550 -> [_ _]
          tunnel: w549 -> [_ w570]
          tunnel: [w564 w567] -> w548
          tunnel: w547 -> [w564 w568]
          tunnel: w542 -> [_ w569]
          frame False {
            n243 = for {
              tunnel: string[] ["SM_VOLTAGE", "MERLIN_VALUE", "DCVoltage", "DCCurrent"] ("State Array Out") -> [w566] mode=indexing
              tunnel: [w565] -> w562 mode=indexing
              n244 = call-poly "VariableManager.vi"("Tag"=w566) -> ("Value out"=w565:dbl)  [unwired: 6 in, 4 out]
            }
            n245 = Index Array(array=w562, index #1=0 ("index")) -> (element #1=→"Source Meter Voltage":dbl, element #2=→"Merlin Voltage":dbl, element #3=→"Agilent Voltage":dbl, element #4=→"Agilent Current":dbl)  [unwired: 3 in]
          }
          frame True {
            n246 = case shown="\"Script\"" w571 {
              tunnel: w570 -> [_ _ _]
              tunnel: w569 -> [_ w575 w582]
              tunnel: w568 -> [w574 w577 w584]
              tunnel: [w572 w576 w583] -> w567
              frame "Voltage Vs Time", Default {
                n247 = Build Array (concatenate)(w574, "accumVTValues" ("String")) -> (w572:string[])
              }
              frame "Voltage Vs Wavelength" {
                n248 = case shown="False" w575 {
                  tunnel: w577 -> [w580 w581]
                  tunnel: [w579 w581] -> w576
                  frame False {
                    n249 = Build Array (concatenate)(w580, "updateSweepGraph" ("String")) -> (w579:string[])
                  }
                  frame True {
                  }
                }
              }
              frame "Script" {
                n250 = case shown="True" w582 {
                  tunnel: w584 -> [w586 w588]
                  tunnel: [w585 w588] -> w583
                  frame False {
                    n251 = Build Array (concatenate)(w586, "executeScript" ("String")) -> (w585:string[])
                  }
                  frame True {
                  }
                }
              }
            }
          }
        }
        n252 = call-poly "VariableManager.vi"("Tag"="measurinWave") -> ("Value out"=→"Measuring Wavelength":dbl)  [unwired: 6 in, 4 out]
      }
      frame "accumVTValues" {
        n253 = Unbundle By Name(w596) -> ("startTime"=w602:u32, "SMVolt"=w598:dbl[], "Test Mode"=w593:enum16{"Time Mode", "dV/dt Mode"})
        n254 = local read "Test Time"() -> (w601:dbl)
        n255 = Tick Count (ms)() -> (millisecond timer value=w603:u32)
        n256 = Subtract(x=w603, y=w602) -> (x-y=w604:u32)
        n257 = call-poly "VariableManager.vi"("Tag"="SM_VOLTAGE") -> ("Value out"=w589:dbl)  [unwired: 6 in, 4 out]
        n258 = Divide(x=w604, y=u32 1000) -> (x/y=w597:dbl)
        n259 = Subtract(x=w601, y=w597) -> (x-y=w600:dbl)
        n260 = Build Array (concatenate)(w598, w589) -> (w594:dbl[])
        n261 = Bundle By Name(cluster=w596, "SMVolt"=w594) -> (w595:T6)
        n262 = case shown="\"dV/dt Mode\"" w593 {
          tunnel: w600 -> [w609 _]
          frame "Time Mode", Default {
            n263 = local write "Time Remaining"(w609) -> ()
          }
          frame "dV/dt Mode" {
            n264 = local write "Time Remaining"(0.0 ("Time Remaining")) -> ()
          }
        }
        n265 = Build Array (concatenate)(w591, "updateVTGraph" ("String")) -> (w590:string[])
      }
      frame "updateVTGraph" {
        n266 = Unbundle By Name(w625) -> ("graphUpdate"=w616:u32, "startTime"=w615:u32, "SMVolt"=w624:dbl[], "lastVoltage"=w623:dbl)
        n267 = Tick Count (ms)() -> (millisecond timer value=w617:u32)
        n268 = Subtract(x=w617, y=w615) -> (x-y=w618:u32)
        n269 = Subtract(x=w617, y=w616) -> (x-y=w621:u32)
        n270 = Divide(x=w618, y=u32 1000) -> (x/y=w613:dbl)
        n271 = Greater Or Equal?(x=w621, y="Log Interval") -> (x >= y?=w614:bool)
        n272 = case shown="True" w614 {
          tunnel: w625 -> [w630 w643]
          tunnel: w624 -> [_ w642]
          tunnel: w623 -> [_ w641]
          tunnel: [w630 w638] -> w622
          tunnel: w613 -> [_ w635]
          tunnel: w612 -> [w629 w633]
          tunnel: [w629 w632] -> w611
          frame False {
          }
          frame True {
            w637 = dbl[] [] ("time")
            n273 = call "getAvarageVoltageForInterval.vi"("lastVal"=w641, "voltages"=w642) -> ("avarage"=w634:dbl)  [unwired: 9 in]
            n274 = local write "Source Meter Voltage"(w634) -> ()
            n275 = local read "VTGraph"() -> (w639:cluster{dbl[], dbl[]})
            n276 = Unbundle(w639) -> (w647:dbl[], w646:dbl[])
            n277 = Tick Count (ms)() -> (millisecond timer value=w636:u32)
            n278 = Build Array (concatenate)(w633, "checkForVTAbort" ("String")) -> (w632:string[])
            n279 = Build Array (concatenate)(w647, w635) -> (w645:dbl[])
            n280 = Build Array (concatenate)(w646, w634) -> (w644:dbl[])
            n281 = Bundle By Name(cluster=w643, "time"=w637, "SMVolt"=w637, "graphUpdate"=w636, "lastVoltage"=w634) -> (w638:T6)
            n282 = Bundle(w645, w644) -> (→"VTGraph":cluster{dbl[], dbl[]})  [unwired: 1 in]
          }
        }
      }
      frame "checkForVTAbort" {
        n283 = Unbundle By Name(w654) -> ("Test Mode"=w655:enum16{"Time Mode", "dV/dt Mode"})  [unwired: 1 out]
        n284 = case shown="\"Time Mode\", Default" w655 {
          tunnel: w654 -> [w660 w676]
          tunnel: [w660 w676] -> w653
          tunnel: [w659 w669] -> w651
          frame "Time Mode", Default {
            n285 = local read "Time Remaining"() -> (w661:dbl)
            n286 = Greater Or Equal To 0?(x=w661) -> (x >= 0?=w659:bool)
          }
          frame "dV/dt Mode" {
            n287 = local read "VTGraph"() -> (w668:cluster{dbl[], dbl[]})
            n288 = local read "Log Interval"() -> (w662:u32)
            n289 = local read "Locked Time"() -> (w670:dbl)
            n290 = Unbundle(w668) -> (w666:dbl[], w667:dbl[])
            n291 = call "getdVbydt.vi"("times"=w666, "voltages"=w667) -> ("dV/dT"=w665:dbl)  [unwired: 7 in, 2 out]
            "dV/dt" <- w665
            n292 = Divide(x=w662, y=1000.0 ("x")) -> (x/y=w664:dbl)
            n293 = Less Or Equal?(x=w665, y="Target dV/dt") -> (x <= y?=w675:bool)
            n294 = Add(x=w664, y=w670) -> (x+y=w674:dbl)
            n295 = case shown="True" w675 {
              tunnel: [0.0 ("Locked Time") w678] -> w672
              tunnel: w674 -> [_ w678]
              frame False {
              }
              frame True {
              }
            }
            "Locked Time" <- w672
            n296 = Greater Or Equal?(x="Lock In time", y=w672) -> (x >= y?=w669:bool)
          }
        }
        n297 = Build Array (concatenate)(w650, "checkNextTest" ("String")) -> (w649:string[])
        n298 = Bundle By Name(cluster=w653, "run?"=w651) -> (w652:T6)
      }
      frame "checkNextTest" {
        n299 = Unbundle By Name(w687) -> ("run?"=w686:bool, "tab"=w680:T1)
        n300 = Equal?(x=w680, y="Perform Test After") -> (x = y?=w685:bool)
        n301 = Build Array (concatenate)(w682, "onStartClicked" ("String")) -> (w683:string[])
        n302 = case shown="False" w686 {
          tunnel: w685 -> [w693 _]
          tunnel: w682 -> [w697 w698]
          tunnel: [w696 w698] -> w684
          tunnel: w683 -> [w695 _]
          tunnel: w680 -> [w692 _]
          tunnel: "Perform Test After" -> [w694 _]
          frame False {
            n303 = Select(t=w697, s=w693, f=w695) -> (s? t:f=w696:string[])
            n304 = Select(t=w692, s=w693, f=w694) -> (s? t:f=w691:T1)
            n305 = local write "tab"(w691) -> ()
          }
          frame True {
          }
        }
      }
      frame "updateSweepGraph" {
        n306 = Unbundle By Name(w708) -> ("graphUpdate"=w711:u32)
        n307 = Tick Count (ms)() -> (millisecond timer value=w699:u32)
        n308 = Subtract(x=w699, y=w711) -> (x-y=w712:u32)
        n309 = Greater Or Equal?(x=w712, y="Settling Time (ms)") -> (x >= y?=w709:bool)
        n310 = for {
          tunnel: string[] ["SM_VOLTAGE", "MERLIN_VALUE"] ("State Array Out") -> [w717] mode=indexing
          tunnel: [w716] -> w703 mode=indexing
          n311 = call-poly "VariableManager.vi"("Tag"=w717) -> ("Value out"=w716:dbl)  [unwired: 6 in, 4 out]
        }
        n312 = Index Array(array=w703, index #1=0 ("index")) -> (element #1=w701:dbl, element #2=w700:dbl)  [unwired: 1 in]
        n313 = case shown="True" w709 {
          tunnel: w708 -> [w746 w755]
          tunnel: [w730 w754] -> w707
          tunnel: w706 -> [w747 w756]
          tunnel: [w728 w756] -> w705
          tunnel: w701 -> [_ w749]
          tunnel: w700 -> [_ w748]
          tunnel: w699 -> [w720 _]
          frame True {
            w729 = dbl[] [] ("SMVolt")
            n314 = local read "Measuring Wavelength"() -> (w738:dbl)
            n315 = local read "sweep"() -> (w745:cluster{dbl[], dbl[]}[])
            n316 = Unbundle By Name(w746) -> ("SMVolt"=w737:dbl[], "MerlinVal"=w736:dbl[])
            n317 = Index Array(array=w745, index #1=0 ("index")) -> (element #1=w743:cluster{dbl[], dbl[]}, element #2=w742:cluster{dbl[], dbl[]})  [unwired: 1 in]
            n318 = Unbundle(w743) -> (w741:dbl[], w740:dbl[])
            n319 = Unbundle(w742) -> (w739:dbl[])  [unwired: 1 out]
            n320 = call "AvarageSamples.vi"("samples"=w737) -> ("Avg"=w735:dbl)  [unwired: 10 in]
            n321 = call "AvarageSamples.vi"("samples"=w736) -> ("Avg"=w734:dbl)  [unwired: 10 in]
            n322 = Build Array (concatenate)(w741, w738) -> (w722:dbl[])
            n323 = Build Array (concatenate)(w740, w735) -> (w719:dbl[])
            n324 = Build Array (concatenate)(w739, w734) -> (w721:dbl[])
            n325 = Build Array (concatenate)(w747, "updateSweep") -> (w728:string[])
            n326 = Bundle(w722, w719) -> (w733:cluster{dbl[], dbl[]})  [unwired: 1 in]
            n327 = Bundle(w722, w721) -> (w732:cluster{dbl[], dbl[]})  [unwired: 1 in]
            n328 = Build Array(w722, w719, dbl[] [] ("element")) -> (w725:dbl[][])
            n329 = Bundle By Name(cluster=w746, "SMVolt"=w729, "MerlinVal"=w729, "graphUpdate"=w720) -> (w730:T6)
            n330 = Number To Fractional String(number=w725, width (-)=i16 7) -> (F-format string=w724:string[][])  [unwired: 2 in]
            n331 = Build Array(w733, w732) -> (→"sweep":cluster{dbl[], dbl[]}[])
            n332 = Transpose 2D Array(2D array=w724) -> (transposed array=w723:string[][])
            n333 = property on="Sweep Results" class="MCListbox (strict)"("ItemNames"=w723) -> ()  [unwired: 2 in, 2 out]
          }
          frame False {
            n334 = Unbundle By Name(w755) -> ("SMVolt"=w753:dbl[], "MerlinVal"=w752:dbl[])
            n335 = Build Array (concatenate)(w753, w749) -> (w751:dbl[])
            n336 = Build Array (concatenate)(w752, w748) -> (w750:dbl[])
            n337 = Bundle By Name(cluster=w755, "SMVolt"=w751, "MerlinVal"=w750) -> (w754:T6)
          }
        }
        n338 = local write "Source Meter Voltage"(w701) -> ()
        n339 = local write "Merlin Voltage"(w700) -> ()
      }
      frame "updateSweep" {
        n340 = Unbundle By Name(w777) -> ("SMVolt"=w775:dbl[], "MerlinVal"=w774:dbl[], "sweepType"=w766:enum16{"ASC", "DESC"}, "From"=w765:dbl)
        n341 = local read "To"() -> (w763:dbl)
        n342 = case shown="\"ASC\"" w766 {
          tunnel: w765 -> [w803 w808]
          tunnel: "Step" -> [w807 w812]
          tunnel: [w806 w811] -> w758
          tunnel: w763 -> [w805 w810]
          tunnel: [w804 w809] -> w762
          tunnel: [w803 w808] -> w759
          frame "DESC" {
            n343 = Subtract(x=w803, y=w807) -> (x-y=w806:dbl)
            n344 = Less Or Equal?(x=w805, y=w803) -> (x <= y?=w804:bool)
          }
          frame "ASC" {
            n345 = Add(x=w808, y=w812) -> (x+y=w811:dbl)
            n346 = Greater Or Equal?(x=w810, y=w808) -> (x >= y?=w809:bool)
          }
        }
        n347 = local read "From"() -> (w757:dbl)
        n348 = case shown="True" w762 {
          tunnel: w760 -> [w799 w802]
          tunnel: [w798 w801] -> w761
          tunnel: w759 -> [_ w800]
          tunnel: w757 -> [w781 _]
          frame False {
            w787 = 0 ("index (row)")
            n349 = local read "sweep"() -> (w795:cluster{dbl[], dbl[]}[])
            n350 = call "setWavelenght.vi"("error in (no error)"=w799, "wavelength"=w781) -> ("error out"=w798:errorcluster)  [unwired: 9 in]
            n351 = property on="Sweep Results" class="MCListbox (strict)"() -> ("ItemNames"=w797:string[][])  [unwired: 2 in, 2 out]
            n352 = Index Array(array=w795, index #1=0 ("index")) -> (element #1=w793:cluster{dbl[], dbl[]}, element #2=w792:cluster{dbl[], dbl[]})  [unwired: 1 in]
            n353 = Unbundle(w793) -> (w790:dbl[], w788:dbl[])
            n354 = Unbundle(w792) -> (w789:dbl[])  [unwired: 1 out]
            n355 = Delete From Array(array=w797, index (row)=w787) -> (array with subset deleted=w796:string[][])  [unwired: 2 in, 1 out]
            n356 = Delete From Array(array=w790, index=w787) -> (array with subset deleted=w786:dbl[])  [unwired: 1 in, 1 out]
            n357 = Delete From Array(array=w788, index=w787) -> (array with subset deleted=w785:dbl[])  [unwired: 1 in, 1 out]
            n358 = Delete From Array(array=w789, index=w787) -> (array with subset deleted=w784:dbl[])  [unwired: 1 in, 1 out]
            n359 = Bundle(w786, w785) -> (w783:cluster{dbl[], dbl[]})  [unwired: 1 in]
            n360 = Bundle(w786, w784) -> (w782:cluster{dbl[], dbl[]})  [unwired: 1 in]
            n361 = property on="Sweep Results" class="MCListbox (strict)"("ItemNames"=w796) -> ()  [unwired: 2 in, 2 out]
            n362 = Build Array(w783, w782) -> (w791:cluster{dbl[], dbl[]}[])
            n363 = local write "sweep"(w791) -> ()
          }
          frame True {
            n364 = call "setWavelenght.vi"("error in (no error)"=w802, "wavelength"=w800) -> ("error out"=w801:errorcluster)  [unwired: 9 in]
          }
        }
        n365 = for {
          tunnel: string[] ["SM_VOLTAGE", "MERLIN_VALUE"] ("State Array Out") -> [w814] mode=indexing
          tunnel: [w813] -> w770 mode=indexing
          n366 = call-poly "VariableManager.vi"("Tag"=w814) -> ("Value out"=w813:dbl)  [unwired: 6 in, 4 out]
        }
        n367 = Index Array(array=w770, index #1=0 ("index")) -> (element #1=w768:dbl, element #2=w767:dbl)  [unwired: 1 in]
        n368 = Build Array (concatenate)(w775, w768) -> (w773:dbl[])
        n369 = Build Array (concatenate)(w774, w767) -> (w772:dbl[])
        n370 = Bundle By Name(cluster=w777, "SMVolt"=w773, "MerlinVal"=w772, "run?"=w762, "From"=w758) -> (w776:T6)
      }
      frame "executeScript" {
        n371 = for {
          tunnel: string[] ["DCVoltage", "DCCurrent", "SM_VOLTAGE"] ("State Array Out") -> [w851] mode=indexing
          tunnel: [w850] -> w827 mode=indexing
          n372 = call-poly "VariableManager.vi"("Tag"=w851) -> ("Value out"=w850:dbl)  [unwired: 6 in, 4 out]
        }
        n373 = Unbundle By Name(w821) -> ("script"=w817:string[][], "lastUpdate"=w829:u32)
        n374 = Index Array(array=w827, index #1=0 ("index")) -> (element #1=w824:dbl, element #2=w825:dbl, element #3=w819:dbl)  [unwired: 2 in]
        n375 = call "executeScript.vi"("script"=w817, "lastUpdate"=w829, "error in (no error)"=w831) -> ("scriptOut"=w816:string[][], "lastUpdate 2"=w820:u32, "error out"=w830:errorcluster)  [unwired: 5 in]
        n376 = local write "Source Meter Voltage"(w819) -> ()
        n377 = local write "Agilent Current"(w825) -> ()
        n378 = local write "Agilent Voltage"(w824) -> ()
        n379 = Empty Array?(array=w816) -> (empty?=w818:bool)
        n380 = Not(x=w818) -> (.not. x?=w815:bool)
        n381 = case shown="False" w815 {
          frame False {
            w844 = 0 ("index (row)")
            n382 = local read "scriptSweep"() -> (w836:cluster{dbl[], dbl[]}[])
            n383 = Index Array(array=w836, index #1=0 ("index")) -> (element #1=w838:cluster{dbl[], dbl[]}, element #2=w839:cluster{dbl[], dbl[]})  [unwired: 1 in]
            n384 = Unbundle(w838) -> (w841:dbl[], w843:dbl[])
            n385 = Unbundle(w839) -> (w842:dbl[])  [unwired: 1 out]
            n386 = Delete From Array(array=w841, index=w844) -> (array with subset deleted=w845:dbl[])  [unwired: 1 in, 1 out]
            n387 = Delete From Array(array=w843, index=w844) -> (array with subset deleted=w846:dbl[])  [unwired: 1 in, 1 out]
            n388 = Delete From Array(array=w842, index=w844) -> (array with subset deleted=w847:dbl[])  [unwired: 1 in, 1 out]
            n389 = Bundle(w845, w846) -> (w848:cluster{dbl[], dbl[]})  [unwired: 1 in]
            n390 = Bundle(w845, w847) -> (w849:cluster{dbl[], dbl[]})  [unwired: 1 in]
            n391 = Build Array(w848, w849) -> (w840:cluster{dbl[], dbl[]}[])
            n392 = local write "scriptSweep"(w840) -> ()
          }
          frame True {
          }
        }
        n393 = Bundle By Name(cluster=w821, "script"=w816, "lastUpdate"=w820, "run?"=w815) -> (w832:T6)
        n394 = Build Array (concatenate)(w835, "updateScriptGraph" ("String")) -> (w823:string[])
      }
      frame "updateScriptGraph" {
        n395 = Unbundle By Name(w860) -> ("startTime"=w864:u32, "time"=w858:dbl[], "SMVolt"=w857:dbl[], "graphUpdate"=w852:u32)
        n396 = call-poly "VariableManager.vi"("Tag"="SM_VOLTAGE" ("String")) -> ("Value out"=w854:dbl)  [unwired: 6 in, 4 out]
        n397 = Tick Count (ms)() -> (millisecond timer value=w853:u32)
        n398 = Subtract(x=w853, y=w852) -> (x-y=w863:u32)
        n399 = Subtract(x=w853, y=w864) -> (x-y=w866:u32)
        n400 = Greater Or Equal?(x=w863, y="Script Avg Interval") -> (x >= y?=w861:bool)
        n401 = Divide(x=w866, y=u32 1000) -> (x/y=w856:dbl)
        n402 = case shown="True" w861 {
          tunnel: w858 -> [w878 _]
          tunnel: w857 -> [w877 w889]
          tunnel: w856 -> [w876 w885]
          tunnel: w854 -> [w875 w883]
          tunnel: w860 -> [w874 w888]
          tunnel: [w873 w887] -> w859
          tunnel: w853 -> [_ w886]
          frame False {
            n403 = Build Array (concatenate)(w878, w876) -> (w872:dbl[])
            n404 = Build Array (concatenate)(w877, w875) -> (w871:dbl[])
            n405 = Bundle By Name(cluster=w874, "time"=w872, "SMVolt"=w871) -> (w873:T6)
          }
          frame True {
            w881 = dbl[] []
            # "smV/Time\nmerlinV/wavelen\nsmV/wavelen"
            n406 = local read "scriptGraph"() -> (w880:cluster{dbl[], dbl[]})
            n407 = Build Array (concatenate)(w889, w883) -> (w884:dbl[])
            n408 = Unbundle(w880) -> (w893:dbl[], w890:dbl[])
            n409 = call "AvarageSamples.vi"("samples"=w884) -> ("Avg"=w882:dbl)  [unwired: 10 in]
            n410 = Build Array (concatenate)(w893, w885) -> (w892:dbl[])
            n411 = Build Array (concatenate)(w890, w882) -> (w891:dbl[])
            n412 = Bundle By Name(cluster=w888, "graphUpdate"=w886, "time"=w881, "SMVolt"=w881) -> (w887:T6)
            n413 = Bundle(cluster=w880, w892, w891) -> (→"scriptGraph":cluster{dbl[], dbl[]})
          }
        }
      }
      frame "---------------Below are Error Handling VIs---------------" {
      }
      frame "Error" {
        n414 = Call Chain() -> (call chain=w909:string[])
        n415 = for {
          tunnel: w909 -> [w917] mode=indexing
          shift-right: [w915] -> w906
          shift-left: "" -> [w918]
          n416 = Concatenate Strings(w918, w917, " -> ") -> (w915:string)
        }
        n417 = Unbundle By Name(w902) -> ("code"=w904:i32, "source"=w903:string)
        n418 = Match Pattern(string=w903, regular expression=":") -> (before substring=w907:string, after substring=w911:string)  [unwired: 1 in, 2 out]
        n419 = Format Into String(format string="Error Occured In\"%s\" state of \"%s\" VI\nError Code: %d\nError Description: \"%s\"", w907, w906, w904, w911) -> (resulting string=w910:string)  [unwired: 2 in, 1 out]
        n420 = One Button Dialog(message=w910) -> ()  [unwired: 1 in, 1 out]
      }
    }
    n421 = Equal?(x="Exit", y=w14) -> (x = y?=w21:bool)
    "Quit" <- w21
    n422 = call "Error Handler.vi"("Current State"=w18, "error in (no error)"=w15, "Msg Queue In"=w19) -> ("error out"=w16:errorcluster, "Msg Queue Out"=w20:string[])  [unwired: 7 in]
  }
  "error out" <- w5
  n423 = property class="App"(error in=w5) -> ("App.Kind"=w4:T5)  [unwired: 1 in, 2 out]
  n424 = Equal?(x=w4, y=T5."Run Time System") -> (x = y?=w2:bool)
  n425 = Quit LabVIEW(quit? (T)=w2) -> ()
